vi "NI6071E.evt call Start DAQ.vi"(0 "i ref in":refnum<vi>, 2 "Client":string, 3 "Client timeout (10000)":i32=10000, 4 "NI6071E Start":T1={"scan rate (40000 scans/sec)"=1.0, "trigger type (analog)"=enum."analog", "edge or slope \n(rising)"=enum."falling", "number of buffers to acquire (1)"=1, "analog chan (PFI0) & level (2.00)"={"trigger channel (empty)"="PFI0", "level (0.0)"=2.0}, "[additional trig params]"={"hysteresis (0.0)"=0.0, "coupling (no change:0)"=enum."no change", "delay (0 sec)"=0.0, "skip count (0)"=0, "time limit (0 sec)"=0.0}} {"[additional trig params]"."time limit (0 sec)" format="%0.2f"; "[additional trig params]"."delay (0 sec)" format="%0.2f"; "[additional trig params]"."hysteresis (0.0)" format="%0.2f"; "analog chan (PFI0) & level (2.00)"."level (0.0)" format="%0.2f"; "scan rate (40000 scans/sec)" format="%0.2f"}, 5 "error in":errorcluster) -> (14 "i ref out":refnum<vi>, 19 "error out":errorcluster)   [LabVIEW 2014, in "NI6071E.lvlib"]
doc: "This VI asks for an event by a simple call"
uses:
  NI6071E.lvlib
  NI6071ECommand.ctl
  NI6071EStart.ctl
  CSCore/CSSystem/CoreLib/CoreLib.string 2 byte array.vi
  CSCore/CSSystem/CoreLib/CoreLib.int 2 byte array.vi
  CSCore/BaseProcess/BaseProcess.lvlib
  CSCore/CSSystem/CoreLib/CoreLib.lvlib
panel:
  in  "NI6071E Command":T2=enum."StartDAQ"
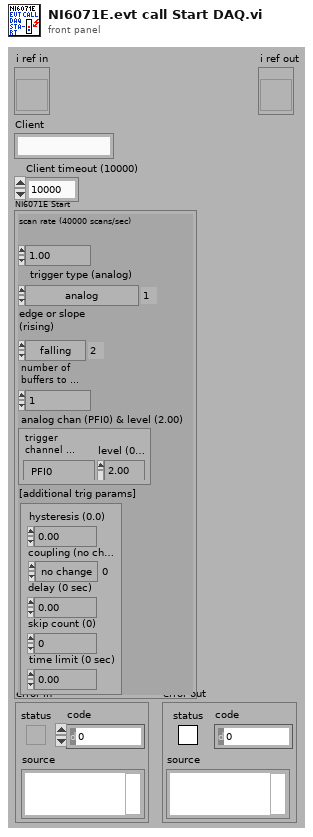
[diagram p1: front panel]
types:
  T1 = typedef "NI6071E.lvlib/NI6071EStart.ctl" = cluster{"scan rate (40000 scans/sec)":sgl, "trigger type (analog)":enum16{"no trigger", "analog", "digital A", "digital A & B", "scan clock gate"}, "edge or slope \n(rising)":enum16{"no change", "rising", "falling"}, "number of buffers to acquire (1)":i32, "analog chan (PFI0) & level (2.00)":cluster{"trigger channel (empty)":string, "level (0.0)":sgl}, "[additional trig params]":cluster{"hysteresis (0.0)":sgl, "coupling (no change:0)":enum16{"no change", "DC", "AC"}, "delay (0 sec)":sgl, "skip count (0)":i32, "time limit (0 sec)":sgl}}
  T2 = typedef "NI6071E.lvlib/NI6071ECommand.ctl" = enum16{"Ping", "Reset", "ConfigureDAQ", "StartDAQ", "StopDAQ", "GetDAQStatus", "ReadData", "SaveData", "CloseConnection"}
  T3 = typedef "CoreDefs.rawDataType.ctl" = i8[]
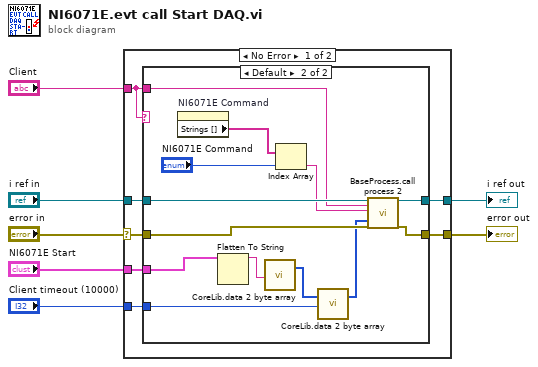
[diagram p0: block diagram]
diagram:
  n1 = case shown="No Error" "error in" {
    selector: "error in" -> [w10 w30]
    tunnel: [w9 w30] -> w7
    tunnel: "i ref in" -> [w14 w31]
    tunnel: "Client" -> [w8 _]
    tunnel: [w13 w31] -> w4
    tunnel: "NI6071E Start" -> [w12 _]
    tunnel: "Client timeout (10000)" -> [w11 _]
    frame No Error {
      n2 = case shown="Default" w8 {
        tunnel: w14 -> [w16 w29]
        tunnel: w8 -> [_ w28]
        tunnel: [w16 w27] -> w13
        tunnel: w12 -> [_ w26]
        tunnel: w11 -> [_ w25]
        tunnel: w10 -> [w15 w24]
        tunnel: [w15 w17] -> w9
        frame "N/A" {
        }
        frame Default {
          n3 = property on="NI6071E Command" class="Enum (strict)"() -> ("Strings []"=w22:string[])  [unwired: 2 in, 2 out]
          n4 = Flatten To String(anything=w26) -> (data string=w20:string)  [unwired: 3 in, 2 out]
          n5 = call-poly "CoreLib.data 2 byte array.vi"("string"=w20) -> ("byteArray out"=w18:T3)  [unwired: 18 in]
          n6 = Index Array(array=w22, index="NI6071E Command") -> (element=w21:string)
          n7 = call-poly "CoreLib.data 2 byte array.vi"("byteArray"=w18, "i32"=w25) -> ("byteArray out"=w19:T3)  [unwired: 17 in]
          n8 = call "BaseProcess.call process 2.vi"("i ref in"=w29, "Object"=w28, "Selector"=w21, "Data"=w19, "error in (no error)"=w24) -> ("i ref out"=w27:refnum<vi>, "error out"=w17:errorcluster)  [unwired: 13 in]
        }
      }
    }
    frame Error {
    }
  }
  "error out" <- w7
  "i ref out" <- w4
